vi "题目1.vi"() -> ()   [LabVIEW 2017]
panel:
  out "波形图 2":dbl[](graph)
  in  "滑动杆 2":dbl(slide) scale=0.0..10.0
  in  "滑动杆":dbl(slide) scale=0.0..10.0
  out "波形图":dbl[](graph)
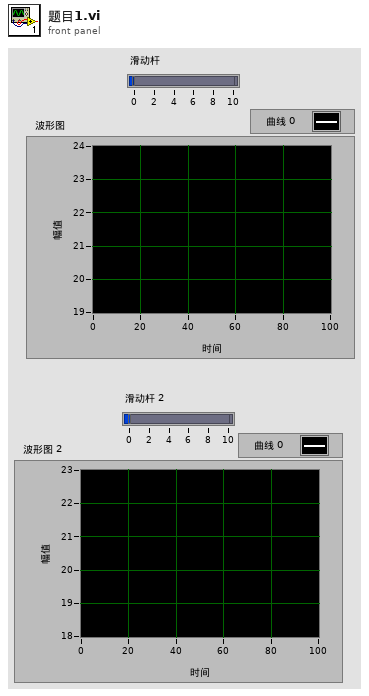
[diagram p1: front panel]
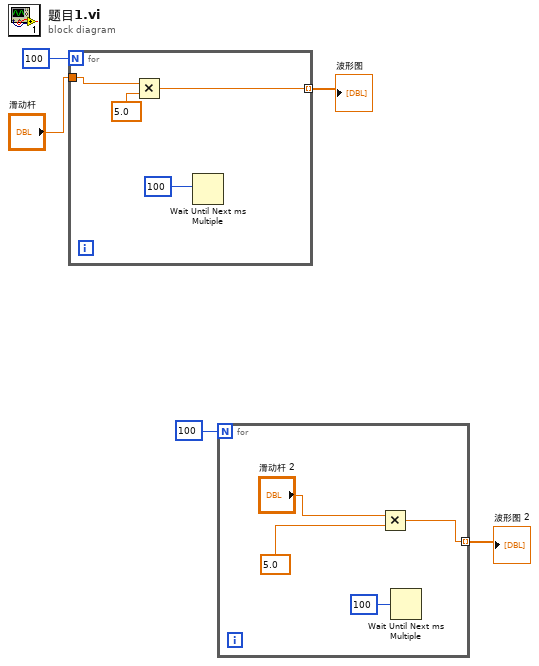
[diagram p0: block diagram]
diagram:
  n1 = for {
    N: 100 -> [_]
    tunnel: "滑动杆" -> [w9]
    tunnel: [w7] -> w3 mode=indexing
    n2 = Multiply(x=w9, y=5.0) -> (x*y=w7:dbl)
    n3 = Wait Until Next ms Multiple(millisecond multiple=100) -> ()  [unwired: 1 out]
  }
  "波形图" <- w3
  n4 = for {
    N: 100 -> [_]
    tunnel: [w10] -> w1 mode=indexing
    n5 = Multiply(x="滑动杆 2", y=5.0) -> (x*y=w10:dbl)
    n6 = Wait Until Next ms Multiple(millisecond multiple=100) -> ()  [unwired: 1 out]
  }
  "波形图 2" <- w1
